vi "Create Series Graph Data.vi"(8 "error in":errorcluster, 9 "Image Index":u32, 10 "Images":refnum<queue>, 11 "Graph with Series View":refnum<class "Graph with Series View.lvclass">) -> (0 "error out":errorcluster, 1 "Cursor Z U16":u16[](array[numeric]), 2 "U16":u16[][](array[numeric]), 4 "Cursor Row Data U16":cluster{"Array":u16[], "U16":u16[]}, 6 "Cursor Col Data U16":cluster{"U16":u16[], "Array":u16[]})   [LabVIEW 2025, in "Graph with Series View.lvclass"]
uses:
  Graph with Series View.lvclass
  HAL/Source/Typedefs/Generic Image/Generic Image.lvclass
  Base Graph/Base Graph.lvclass/Base Graph.ctl
  Base Graph/Base Graph.lvclass
  Detail Graph/Graph with Section Views.lvclass
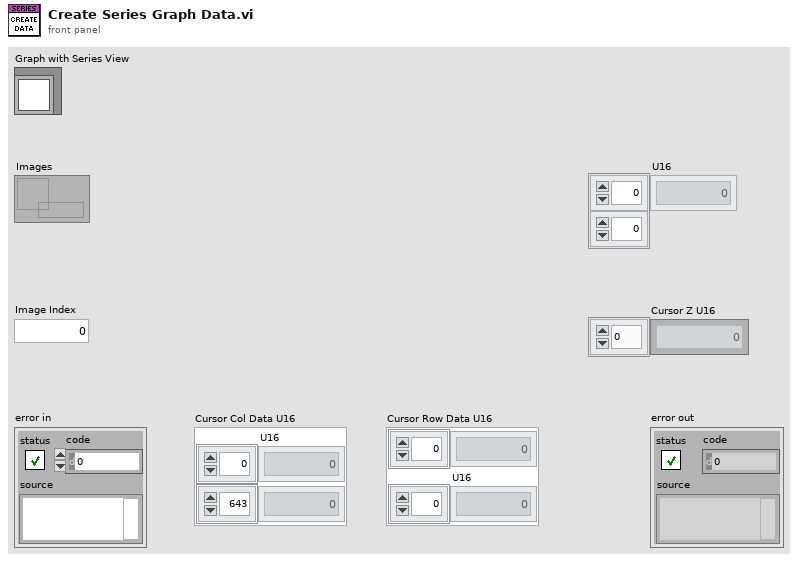
[diagram p1: front panel]
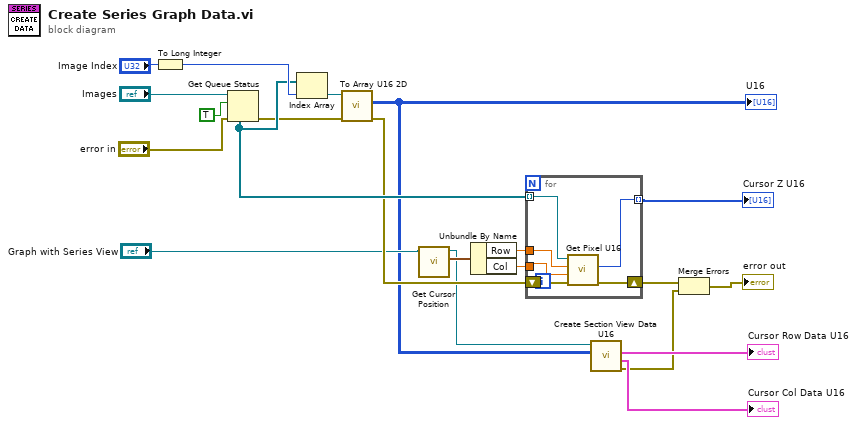
[diagram p0: block diagram]
diagram:
  n1 = To Long Integer(number="Image Index") -> (32bit integer=w18:i32)
  n2 = Get Queue Status(queue="Images", return elements? (F)=TRUE, error in (no error)="error in") -> (error out=w9:errorcluster, elements=w17:refnum<class "Generic Image.lvclass">[])  [unwired: 6 out]
  n3 = Index Array(array=w17, index=w18) -> (element=w16:refnum<class "Generic Image.lvclass">)
  n4 = call "To Array U16 2D.vi"("error in"=w9, "Generic Image in"=w16) -> ("error out"=w10:errorcluster, "U16"=w1:u16[][])  [unwired: 7 in, 1 out]
  "U16" <- w1
  n5 = call "Get Cursor Position.vi"("Base Graph in"="Graph with Series View") -> ("Cursor Position"=w15:cluster{"Col":dbl, "Row":dbl}, "Base Graph out"=w2:refnum<class "Graph with Series View.lvclass">)  [unwired: 9 in]
  n6 = Unbundle By Name(w15) -> ("Row"=w12:dbl, "Col"=w11:dbl)
  n7 = for {
    tunnel: w17 -> [w27] mode=indexing
    tunnel: w12 -> [w23]
    tunnel: w11 -> [w22]
    shift-right: [w25] -> w14
    shift-left: w10 -> [w26]
    tunnel: [w24] -> w13 mode=indexing
    n8 = call-dynamic "Get Pixel U16.vi"("error in"=w26, "col"=w22, "row"=w23, "Generic Image in"=w27) -> ("error out"=w25:errorcluster, "Pixel"=w24:u16)  [unwired: 6 in]
  }
  "Cursor Z U16" <- w13
  n9 = call "Create Section View Data U16.vi"("Image U16"=w1, "Graph with Section Views in"=w2) -> ("error out"=w3:errorcluster, "Cursor Column Data"=→"Cursor Col Data U16":cluster{"Image U16":u16[], "Array":u16[]}, "Cursor Row Data"=→"Cursor Row Data U16":cluster{"Array":u16[], "Image U16":u16[]})  [unwired: 7 in]
  n10 = Merge Errors(w14, w3) -> (→"error out":errorcluster)
